vi "8.1 форма проверки натекания.vi"() -> ()   [LabVIEW 2016, in "Library.lvlib"]
uses:
  Granule-2000AT/PC/Library.lvlib
  <vilib>/Utility/file.llb/Write To Spreadsheet File (string).vi
panel:
  in  "Reset":bool
  out "Elapsed Time (s)":dbl
  out "Time has Elapsed":bool
  in  "закрыть форму":bool
  in  "array_file":string[][](array[string])
  out "Величина течи\n(torr*mkL/sec)":string caption="Вакуум в камере\nPT2 (torr)"
  out "Время цикла (sec)":string caption="Вакуум в камере\nPT2 (torr)"
  out "Время завершения проверки":string caption="Вакуум в камере\nPT2 (torr)"
  out "Время запуска проверки":string caption="Вакуум в камере\nPT2 (torr)"
  in  "stop":bool
  out "выполнить проверку":bool
  out "Vak_out":dbl
  out "условия в норме":bool
  out "param_out":dbl[](array[numeric])
  in  "выполнить проверку натекания":bool
  in  "задать время проверки":bool
  in  "задать конечный вакуум":bool
  in  "задать начальный вакуум":bool
  out "Время проверки (sec)":string caption="Вакуум в камере\nPT2 (torr)"
  out "Конечный вакуум (torr)":string caption="Вакуум в камере\nPT2 (torr)"
  out "Начальный вакуум (torr)":string caption="Вакуум в камере\nPT2 (torr)"
  out "Вакуум в камере (torr)":string caption="Вакуум в камере\nPT2 (torr)"
  out "XY Graph":cluster{"Elapsed Time (s)":dbl, "Vak_out":dbl}[](graph)
  in  "Array":cluster{"Elapsed Time (s)":dbl, "Vak_out":dbl}[](array[cluster])
  in  "PT1":dbl
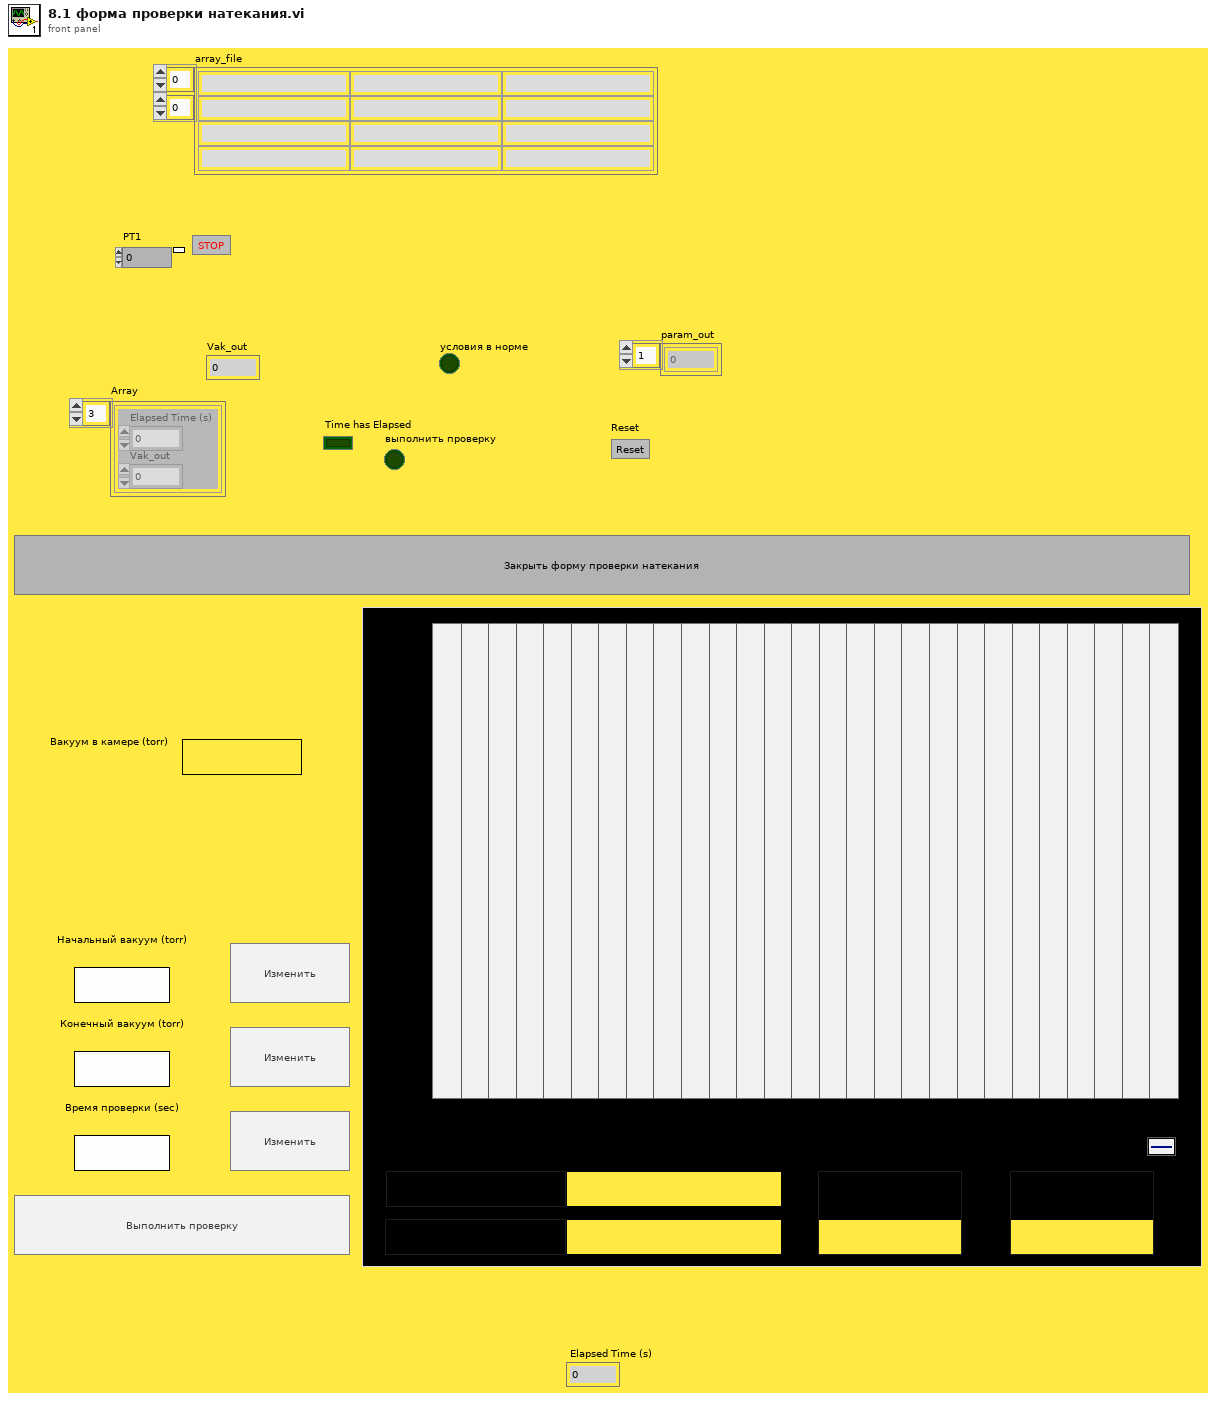
[diagram p1: front panel]
types:
  T1 = enum8{"Enabled", "Disabled", "Disabled and Grayed Out"}
  T2 = cluster{"Начало проверки":string, "Завершение проверки":string, "Время проверки (sec)":string, "Величина течи\n(torr*mkL/sec)":string}
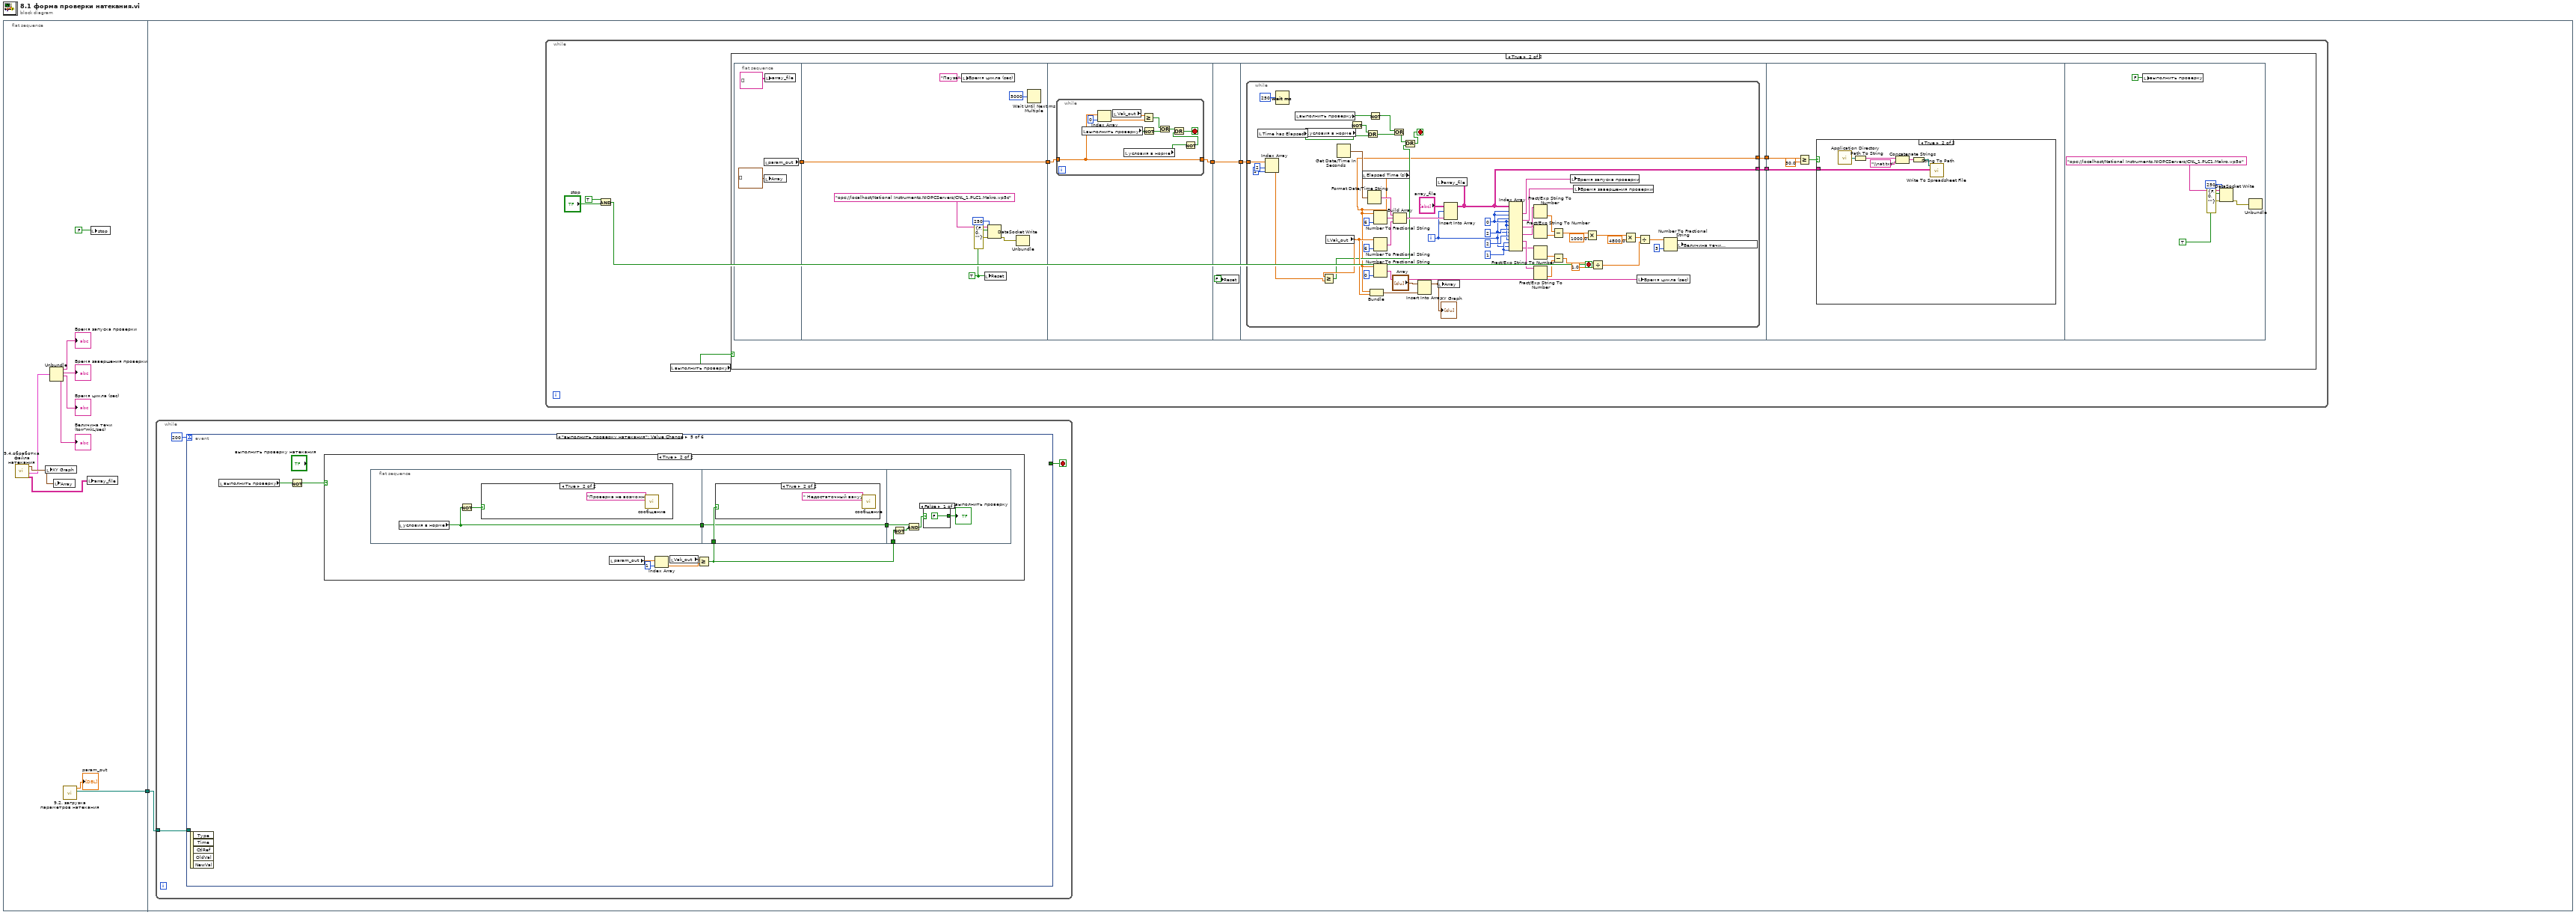
[diagram p0: block diagram]
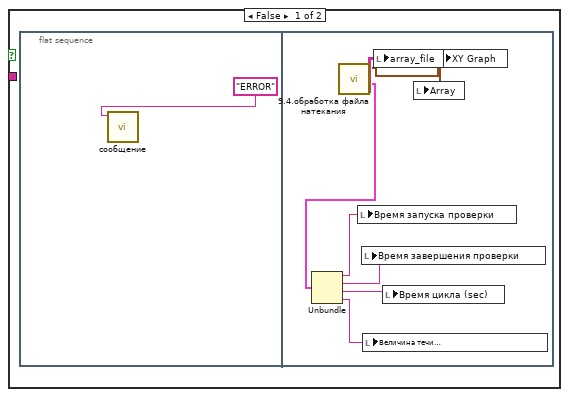
[diagram p3: hidden frame]
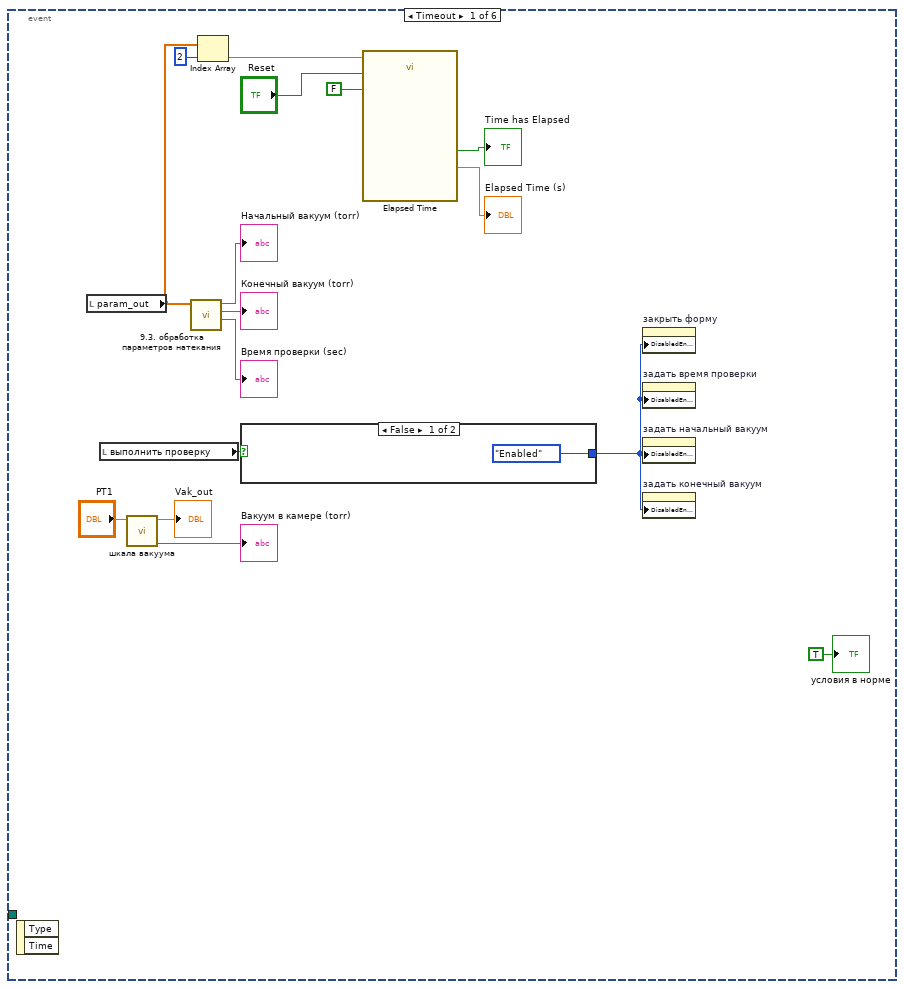
[diagram p4: hidden frame]
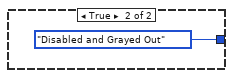
[diagram p5: hidden frame]
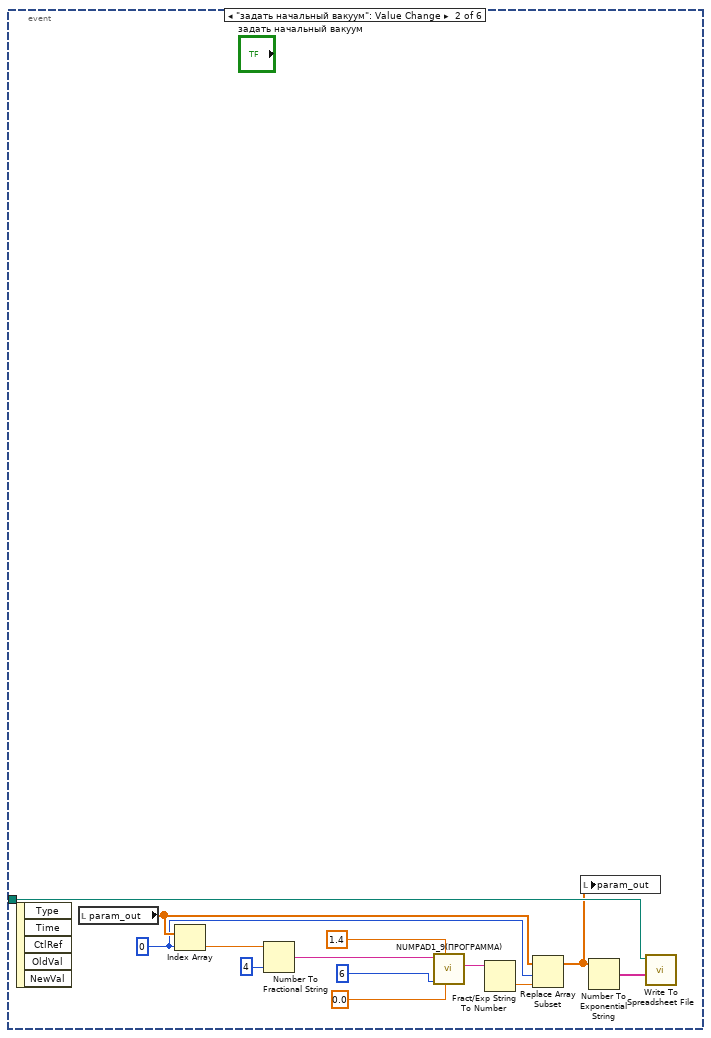
[diagram p6: hidden frame]
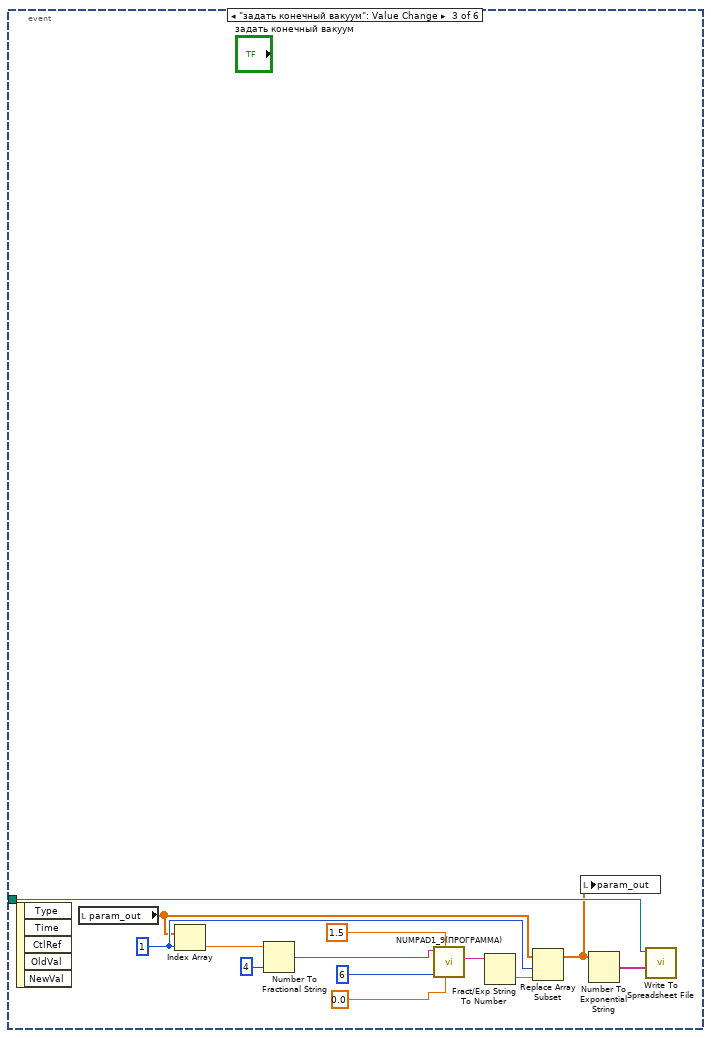
[diagram p7: hidden frame]
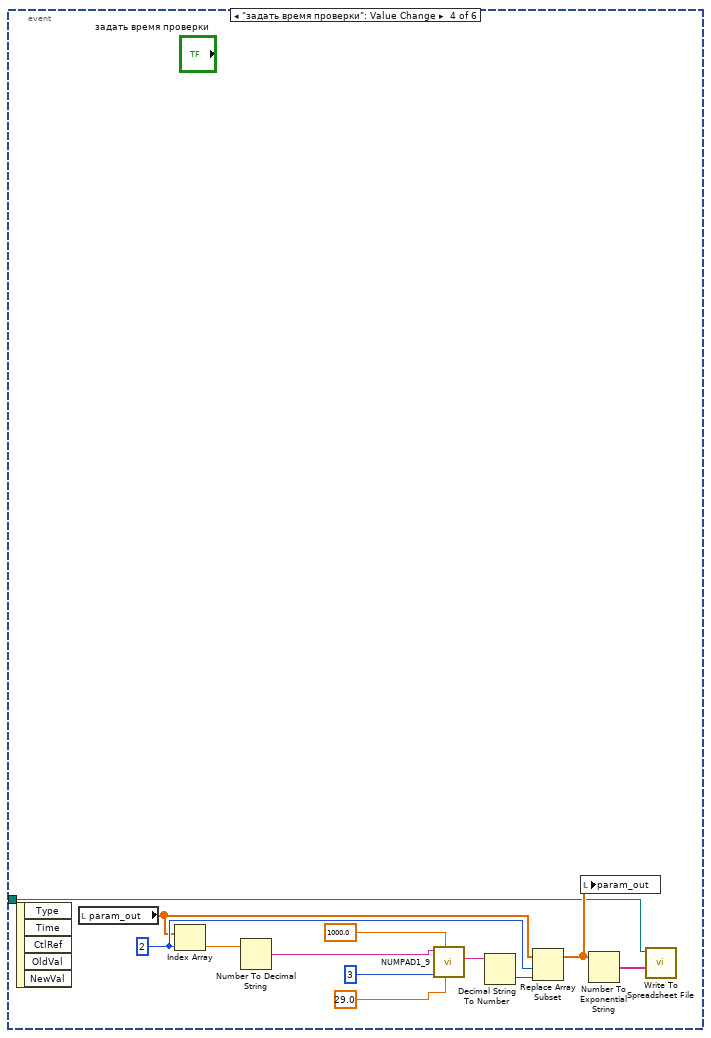
[diagram p8: hidden frame]
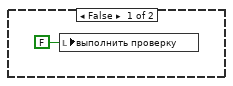
[diagram p9: hidden frame]
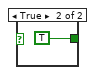
[diagram p12: hidden frame]
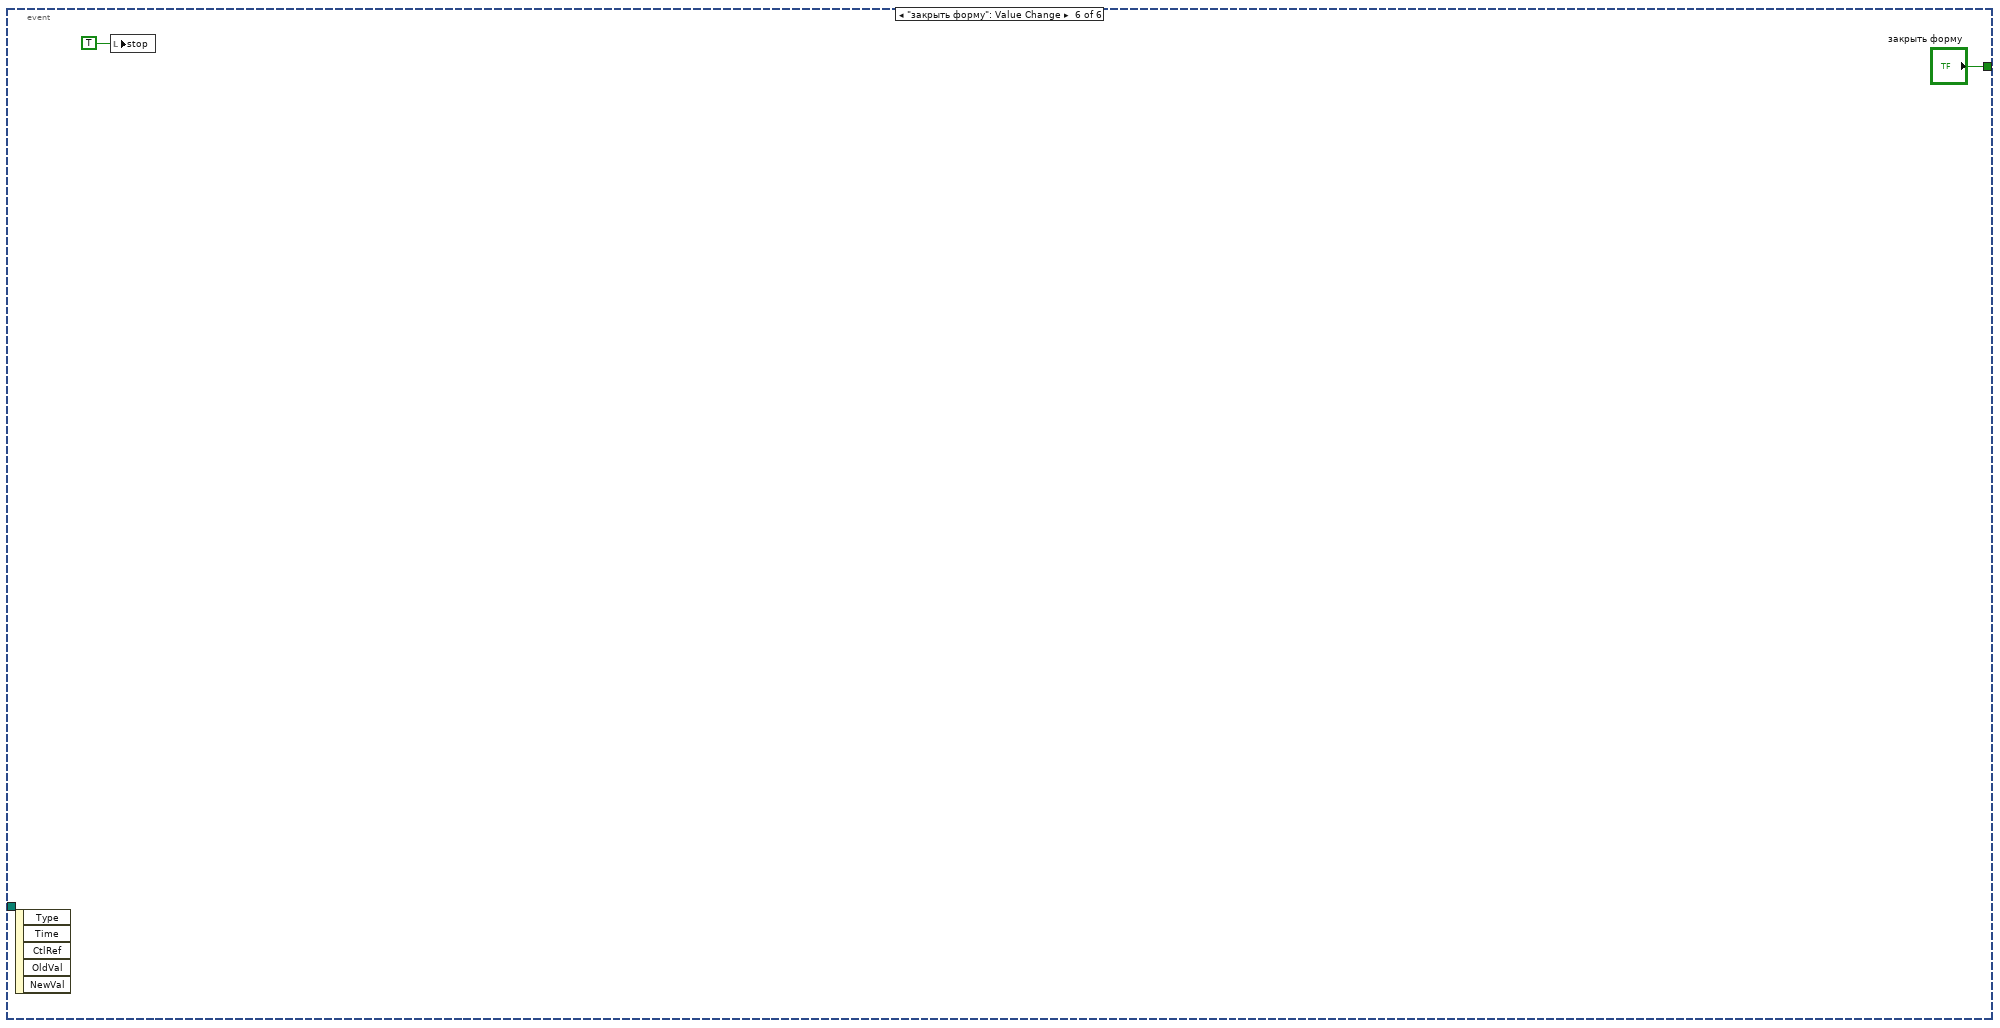
[diagram p13: hidden frame]
diagram:
  n1 = flat-sequence {
    tunnel: [w10] -> w1
    tunnel: w1 -> [w12]
    frame #0 {
      n2 = call "9.4.обработка файла натекания.vi"() -> ("all rows"=w7:string[][], "output cluster"=w6:T2, "array_graph out"=w8:cluster{"String":dbl, "String":dbl}[])  [unwired: 8 in, 1 out]
      n3 = local write "XY Graph"(w8) -> ()
      n4 = Unbundle(w6) -> ("Начало проверки"=→"Время запуска проверки":string, "Завершение проверки"=→"Время завершения проверки":string, "Время проверки (sec)"=→"Время цикла (sec)":string, "Величина течи\n(torr*mkL/sec)"=→"Величина течи\n(torr*mkL/sec)":string)
      n5 = local write "Array"(w8) -> ()
      n6 = call "9.2. загрузка параметров натекания.vi"() -> ("path param"=w10:path, "param_out"=→"param_out":dbl[])  [unwired: 10 in]
      n7 = local write "array_file"(w7) -> ()
      n8 = local write "stop"(FALSE ("stop")) -> ()
    }
    frame #1 {
      n9 = while {
        tunnel: w12 -> [w132]
        stop <- w133 stop-if-true
        n10 = event shown="[4] \"выполнить проверку натекания\": Value Change" {
          selector: _ -> [_ _ _ _ _ _]
          dyn-events: _ -> [_ _ _ _ _ _]
          timeout: 200 -> [_ _ _ _ _ _]
          tunnel: [_ _ _ _ _ "закрыть форму"] -> w133
          tunnel: w132 -> [_ w158 w171 w179 _ _]
          event Timeout {
            n11 = event-data() -> ()  [unwired: 1 in, 2 out]
            n12 = local read "param_out"() -> (w139:dbl[])
            n13 = local read "выполнить проверку"() -> (w144:bool)
            n14 = call "шкала вакуума.vi"("Vak_in"="PT1") -> ("Vak_out_txt"=→"Вакуум в камере (torr)":string, "Vak_out"=→"Vak_out":dbl)  [unwired: 9 in]
            n15 = call "9.3. обработка параметров натекания.vi"("param_out"=w139) -> ("time"=→"Время проверки (sec)":string, "Presure 2"=→"Конечный вакуум (torr)":string, "presure 1"=→"Начальный вакуум (torr)":string)  [unwired: 7 in, 1 out]
            n16 = Index Array(array=w139, index=2) -> (element=w137:dbl)
            n17 = case shown="False" w144 {
              tunnel: [T1."Enabled" ("Disabled") T1."Disabled and Grayed Out" ("Disabled")] -> w143
              frame False {
              }
              frame True {
              }
            }
            n18 = call "Elapsed Time"("Time Target (s)"=w137, "Reset"="Reset", "Auto Reset"=FALSE) -> ("Elapsed Time (s)"=→"Elapsed Time (s)":dbl, "Time has Elapsed"=→"Time has Elapsed":bool)  [unwired: 9 in, 6 out]
            n19 = property on="закрыть форму" class="Bool"("DisabledEnum"=w143) -> ()  [unwired: 2 in, 2 out]
            n20 = property on="задать время проверки" class="Bool"("DisabledEnum"=w143) -> ()  [unwired: 2 in, 2 out]
            n21 = property on="задать начальный вакуум" class="Bool"("DisabledEnum"=w143) -> ()  [unwired: 2 in, 2 out]
            n22 = property on="задать конечный вакуум" class="Bool"("DisabledEnum"=w143) -> ()  [unwired: 2 in, 2 out]
            "условия в норме" <- TRUE ("условия в норме")
          }
          event "задать начальный вакуум": Value Change {
            w159 = 0 ("index")
            n23 = event-data() -> ()  [unwired: 1 in, 5 out]
            n24 = local read "param_out"() -> (w161:dbl[])
            n25 = Index Array(array=w161, index=w159) -> (element=w157:dbl)
            n26 = Number To Fractional String(number=w157, precision (6)=i16 4) -> (F-format string=w156:string)  [unwired: 2 in]
            n27 = call "NUMPAD1_9(ПРОГРАММА).vi"("МИНИМАЛЬНОЕ ЗНАЧЕНИЕ"=0.0, "МАКСИМАЛЬНОЕ ЗНАЧЕНИЕ"=1.4, "ДЛИННА СЛОВА"=i8 6, "ТЕКУЩЕЕ ЗНАЧЕНИЕ"=w156) -> ("НОВОЕ ЗНАЧЕНИЕ"=w163:string)  [unwired: 7 in]
            n28 = Fract/Exp String To Number(string=w163) -> (number=w160:dbl)  [unwired: 3 in, 1 out]
            n29 = Replace Array Subset(array=w161, new element=w160, index=w159) -> (w154:dbl[])
            n30 = local write "param_out"(w154) -> ()
            n31 = Number To Exponential String(number=w154) -> (E-format string=w153:string[])  [unwired: 3 in]
            n32 = call-poly <vilib>:"Write To Spreadsheet File.vi"("1D data"=w153, "file path (dialog if empty)"=w158) -> ()  [unwired: 6 in, 1 out]
          }
          event "задать конечный вакуум": Value Change {
            w173 = 1 ("index")
            n33 = event-data() -> ()  [unwired: 1 in, 5 out]
            n34 = local read "param_out"() -> (w172:dbl[])
            n35 = Index Array(array=w172, index=w173) -> (element=w169:dbl)
            n36 = Number To Fractional String(number=w169, precision (6)=i16 4) -> (F-format string=w170:string)  [unwired: 2 in]
            n37 = call "NUMPAD1_9(ПРОГРАММА).vi"("МИНИМАЛЬНОЕ ЗНАЧЕНИЕ"=0.0, "МАКСИМАЛЬНОЕ ЗНАЧЕНИЕ"=1.5, "ДЛИННА СЛОВА"=i8 6, "ТЕКУЩЕЕ ЗНАЧЕНИЕ"=w170) -> ("НОВОЕ ЗНАЧЕНИЕ"=w176:string)  [unwired: 7 in]
            n38 = Fract/Exp String To Number(string=w176) -> (number=w174:dbl)  [unwired: 3 in, 1 out]
            n39 = Replace Array Subset(array=w172, new element=w174, index=w173) -> (w167:dbl[])
            n40 = local write "param_out"(w167) -> ()
            n41 = Number To Exponential String(number=w167) -> (E-format string=w166:string[])  [unwired: 3 in]
            n42 = call-poly <vilib>:"Write To Spreadsheet File.vi"("1D data"=w166, "file path (dialog if empty)"=w171) -> ()  [unwired: 6 in, 1 out]
          }
          event "задать время проверки": Value Change {
            w190 = 2 ("index")
            n43 = event-data() -> ()  [unwired: 1 in, 5 out]
            n44 = local read "param_out"() -> (w181:dbl[])
            n45 = Index Array(array=w181, index=w190) -> (element=w184:dbl)
            n46 = Number To Decimal String(number=w184) -> (decimal integer string=w185:string)  [unwired: 1 in]
            n47 = call "NUMPAD1_9.vi"("МИНИМАЛЬНОЕ ЗНАЧЕНИЕ"=29.0, "МАКСИМАЛЬНОЕ ЗНАЧЕНИЕ"=1000.0, "ДЛИННА СЛОВА"=i8 3, "ТЕКУЩЕЕ ЗНАЧЕНИЕ"=w185) -> ("НОВОЕ ЗНАЧЕНИЕ"=w183:string)  [unwired: 7 in]
            n48 = Decimal String To Number(string=w183) -> (number=w182:i32)  [unwired: 2 in, 1 out]
            n49 = Replace Array Subset(array=w181, new element=w182, index=w190) -> (w180:dbl[])
            n50 = local write "param_out"(w180) -> ()
            n51 = Number To Exponential String(number=w180) -> (E-format string=w189:string[])  [unwired: 3 in]
            n52 = call-poly <vilib>:"Write To Spreadsheet File.vi"("1D data"=w189, "file path (dialog if empty)"=w179) -> ()  [unwired: 6 in, 1 out]
          }
          event "выполнить проверку натекания": Value Change {
            n53 = event-data() -> ()  [unwired: 1 in, 5 out]
            n54 = local read "выполнить проверку"() -> (w192:bool)
            n55 = Not(x=w192) -> (.not. x?=w191:bool)
            n56 = case shown="True" w191 {
              frame False {
                n57 = local write "выполнить проверку"(FALSE ("выполнить проверку")) -> ()
              }
              frame True {
                n58 = flat-sequence {
                  tunnel: [w201] -> w200
                  tunnel: w194 -> [w205]
                  tunnel: [w204] -> w199
                  tunnel: w200 -> [w204]
                  tunnel: w194 -> [w210]
                  tunnel: w199 -> [w209]
                  frame #0 {
                    n59 = local read "условия в норме"() -> (w201:bool)
                    n60 = Not(x=w201) -> (.not. x?=w202:bool)
                    n61 = case shown="True" w202 {
                      frame False {
                      }
                      frame True {
                        n62 = call "сообщение .vi"("сообщение"="Проверка не возможна") -> ()  [unwired: 11 in]
                      }
                    }
                  }
                  frame #1 {
                    n63 = case shown="True" w205 {
                      frame False {
                      }
                      frame True {
                        n64 = call "сообщение .vi"("сообщение"=" Недостаточный вакуум") -> ()  [unwired: 11 in]
                      }
                    }
                  }
                  frame #2 {
                    n65 = Not(x=w210) -> (.not. x?=w211:bool)
                    n66 = And(x=w209, y=w211) -> (x .and. y?=w208:bool)
                    n67 = case shown="False" w208 {
                      tunnel: [FALSE ("выполнить проверку") TRUE ("выполнить проверку")] -> w207
                      frame False {
                      }
                      frame True {
                      }
                    }
                    "выполнить проверку" <- w207
                  }
                }
                n68 = local read "param_out"() -> (w198:dbl[])
                n69 = Index Array(array=w198, index=1) -> (element=w195:dbl)
                n70 = local read "Vak_out"() -> (w196:dbl)
                n71 = Greater Or Equal?(x=w196, y=w195) -> (x >= y?=w194:bool)
              }
            }
          }
          event "закрыть форму": Value Change {
            n72 = event-data() -> ()  [unwired: 1 in, 5 out]
            n73 = local write "stop"(TRUE ("stop")) -> ()
          }
        }
      }
      n74 = while {
        stop <- w14 stop-if-true
        n75 = And(x=TRUE, y="stop") -> (x .and. y?=w14:bool)
        n76 = local read "выполнить проверку"() -> (w13:bool)
        n77 = case shown="True" w13 {
          frame False {
          }
          frame True {
            n78 = flat-sequence {
              tunnel: [w23] -> w21
              tunnel: [w31] -> w22
              tunnel: w21 -> [w31]
              tunnel: w22 -> [w35]
              tunnel: [w34] -> w18
              tunnel: w18 -> [w48]
              tunnel: [w48] -> w17
              tunnel: w17 -> [w51]
              tunnel: [w50] -> w20
              tunnel: [w49] -> w19
              tunnel: w20 -> [w111]
              tunnel: w19 -> [w108]
              frame #0 {
                n79 = local read "param_out"() -> (w23:dbl[])
                n80 = local write "Array"(cluster{"Elapsed Time (s)":dbl, "Vak_out":dbl}[] [] ("Array")) -> ()
                n81 = local write "array_file"(string[][] [] ("array_file")) -> ()
              }
              frame #1 {
                w29 = TRUE ("Reset")
                n82 = local write "Время цикла (sec)"("Пауза" ("Время проверки (sec)")) -> ()
                n83 = local write "Reset"(w29) -> ()
                n84 = DataSocket Write(8:errorcluster {"status"=FALSE, "code"=0, "source"=""} ("error in (no error)"), 9:250 ("ms timeout (0)"), 10:w29, 11:"opc://localhost/National Instruments.NIOPCServers/CNL_1.PLC1.Makro.vp5c" ("connection in")) -> (0:w27:errorcluster)  [unwired: 2 out]
                n85 = Unbundle(w27) -> ()  [unwired: 3 out]
                n86 = Wait Until Next ms Multiple(millisecond multiple=u32 5000) -> ()  [unwired: 1 out]
              }
              frame #2 {
                n87 = while {
                  tunnel: w35 -> [w45]
                  tunnel: [w45] -> w34
                  stop <- w42 stop-if-true
                  n88 = local read "выполнить проверку"() -> (w40:bool)
                  n89 = Index Array(array=w45, index=0) -> (element=w38:dbl)
                  n90 = local read "Vak_out"() -> (w39:dbl)
                  n91 = local read "условия в норме"() -> (w37:bool)
                  n92 = Greater Or Equal?(x=w39, y=w38) -> (x >= y?=w44:bool)
                  n93 = Not(x=w40) -> (.not. x?=w41:bool)
                  n94 = Or(x=w44, y=w41) -> (x .or. y?=w43:bool)
                  n95 = Not(x=w37) -> (.not. x?=w36:bool)
                  n96 = Or(x=w43, y=w36) -> (x .or. y?=w42:bool)
                }
              }
              frame #3 {
                n97 = local write "Reset"(FALSE ("Reset")) -> ()
              }
              frame #4 {
                n98 = while {
                  tunnel: w51 -> [w69]
                  tunnel: [w55] -> w50
                  tunnel: [w68] -> w49
                  i -> [w80]
                  stop <- w57 stop-if-true
                  w81 = 1 ("disabled index (col)")
                  w82 = 0 ("index (row)")
                  n99 = local read "Time has Elapsed"() -> (w56:bool)
                  n100 = Index Array(array=w69, index #1=2 ("index"), index #2=1 ("index")) -> (element #2=w60:dbl)  [unwired: 1 out]
                  n101 = Wait (ms)(milliseconds to wait=u32 250) -> ()  [unwired: 1 out]
                  n102 = local read "выполнить проверку"() -> (w67:bool)
                  n103 = local read "условия в норме"() -> (w63:bool)
                  n104 = local read "Vak_out"() -> (w62:dbl)
                  n105 = Greater Or Equal?(x=w62, y=w60) -> (x >= y?=w59:bool)
                  n106 = Get Date/Time In Seconds() -> (seconds since 1Jan1904=w100:timestamp)
                  n107 = Not(x=w63) -> (.not. x?=w64:bool)
                  n108 = local read "Elapsed Time (s)"() -> (w55:dbl)
                  n109 = Or(x=w64, y=w56) -> (x .or. y?=w66:bool)
                  n110 = Format Date/Time String(seconds (now)=w100) -> (date/time string=w97:string)  [unwired: 2 in]
                  n111 = Not(x=w67) -> (.not. x?=w65:bool)
                  n112 = Bundle("Elapsed Time (s)"=w55, "Vak_out"=w62) -> (w107:cluster{"Elapsed Time (s)":dbl, "Vak_out":dbl})  [unwired: 1 in]
                  n113 = Number To Fractional String(number=w55, precision (6)=i16 6) -> (F-format string=w96:string)  [unwired: 2 in]
                  n114 = Number To Fractional String(number=w62, precision (6)=i16 6) -> (F-format string=w95:string)  [unwired: 2 in]
                  n115 = Number To Fractional String(number=w55, precision (6)=i16 0) -> (F-format string=w103:string)  [unwired: 2 in]
                  n116 = Or(x=w65, y=w66) -> (x .or. y?=w58:bool)
                  n117 = Build Array(w97, w96, w95) -> (w94:string[])
                  n118 = Or(x=w58, y=w59) -> (x .or. y?=w57:bool)
                  n119 = Insert Into Array(array="Array", new element=w107) -> (w106:cluster{"Elapsed Time (s)":dbl, "Vak_out":dbl}[])  [unwired: 1 in]
                  "XY Graph" <- w106
                  n120 = local write "Array"(w106) -> ()
                  n121 = Insert Into Array(array="array_file", index (row)=w80, new element=w94) -> (w68:string[][])  [unwired: 1 in]
                  n122 = local write "array_file"(w68) -> ()
                  n123 = Index Array(array=w68, index (row) #1=w82, index (col) #1=w82, index (row) #2=w80, index (col) #2=w82, index (row) #3=w82, index (col) #3=2 ("disabled index (col)"), index (row) #4=w80, index (col) #4=2 ("index (col)"), index (row) #5=w82, index (col) #5=w81, index (row) #6=w80, index (col) #6=w81) -> (element #1=w92:string, element #2=w91:string, element #3=w89:string, element #4=w87:string, element #5=w79:string, element #6=w78:string)
                  n124 = Fract/Exp String To Number(string=w87) -> (number=w86:dbl)  [unwired: 3 in, 1 out]
                  n125 = Fract/Exp String To Number(string=w89) -> (number=w85:dbl)  [unwired: 3 in, 1 out]
                  n126 = Fract/Exp String To Number(string=w78) -> (number=w77:dbl)  [unwired: 3 in, 1 out]
                  n127 = Fract/Exp String To Number(string=w79) -> (number=w76:dbl)  [unwired: 3 in, 1 out]
                  n128 = Subtract(x=w86, y=w85) -> (x-y=w84:dbl)
                  n129 = Subtract(x=w77, y=w76) -> (x-y=w54:dbl)
                  n130 = local write "Время запуска проверки"(w92) -> ()
                  n131 = local write "Время завершения проверки"(w91) -> ()
                  n132 = Multiply(x=w84, y=1000.0) -> (x*y=w75:dbl)
                  n133 = Divide(x=w54, y=1.0) -> (x/y=w52:dbl)
                  n134 = Multiply(x=w75, y=4800.0) -> (x*y=w73:dbl)
                  n135 = local write "Время цикла (sec)"(w103) -> ()
                  n136 = Divide(x=w73, y=w52) -> (x/y=w72:dbl)
                  n137 = Number To Fractional String(number=w72, precision (6)=i16 3) -> (F-format string=w70:string)  [unwired: 2 in]
                  n138 = local write "Величина течи\n(torr*mkL/sec)"(w70) -> ()
                }
              }
              frame #5 {
                n139 = Greater Or Equal?(x=w111, y=30.0) -> (x >= y?=w109:bool)
                n140 = case shown="True" w109 {
                  tunnel: w108 -> [_ w125]
                  frame False {
                    n141 = flat-sequence {
                      frame #0 {
                        n142 = call "сообщение .vi"("сообщение"="ERROR") -> ()  [unwired: 11 in]
                      }
                      frame #1 {
                        n143 = call "9.4.обработка файла натекания.vi"() -> ("all rows"=w119:string[][], "output cluster"=w113:T2, "array_graph out"=w118:cluster{"String":dbl, "String":dbl}[])  [unwired: 8 in, 1 out]
                        n144 = Unbundle(w113) -> ("Начало проверки"=w117:string, "Завершение проверки"=w116:string, "Время проверки (sec)"=w115:string, "Величина течи\n(torr*mkL/sec)"=w114:string)
                        n145 = local write "Время запуска проверки"(w117) -> ()
                        n146 = local write "Время завершения проверки"(w116) -> ()
                        n147 = local write "Величина течи\n(torr*mkL/sec)"(w114) -> ()
                        n148 = local write "array_file"(w119) -> ()
                        n149 = local write "Время цикла (sec)"(w115) -> ()
                        n150 = local write "Array"(w118) -> ()
                        n151 = local write "XY Graph"(w118) -> ()
                      }
                    }
                  }
                  frame True {
                    n152 = call <vilib>:"Application Directory.vi"() -> ("Application Directory"=w124:path)
                    n153 = Path To String(path=w124) -> (string=w123:string)
                    n154 = Concatenate Strings(w123, "\\nat.txt" ("string")) -> (w121:string)
                    n155 = String To Path(string=w121) -> (path=w120:path)
                    n156 = call-poly <vilib>:"Write To Spreadsheet File.vi"("2D data"=w125, "file path (dialog if empty)"=w120) -> ()  [unwired: 6 in, 1 out]
                  }
                }
              }
              frame #6 {
                n157 = local write "выполнить проверку"(FALSE ("выполнить проверку")) -> ()
                n158 = DataSocket Write(8:errorcluster {"status"=FALSE, "code"=0, "source"=""} ("error in (no error)"), 9:250 ("ms timeout (0)"), 10:TRUE, 11:"opc://localhost/National Instruments.NIOPCServers/CNL_1.PLC1.Makro.vp5o" ("connection in")) -> (0:w128:errorcluster)  [unwired: 2 out]
                n159 = Unbundle(w128) -> ()  [unwired: 3 out]
              }
            }
          }
        }
      }
    }
  }
